vi "multipart_upload.initialize_upload.vi"() -> ()   [LabVIEW 2020, in "Nominal Client.lvclass"]
uses:
  Nominal Client.lvclass
  <vilib>/addons/_JKI.lib/REST Client/classes/REST Client/REST Client.lvclass
  upload.part_core.vi
  Nominal Client.lvclass/Nominal Client.ctl
  Nominal Client MultiPart Upload/Multipart Upload.lvclass
panel:
  out "output cluster":T1
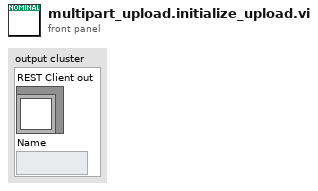
[diagram p1: front panel]
types:
  T1 = cluster{"REST Client out":refnum<class "REST Client.lvclass">, "Name":string}
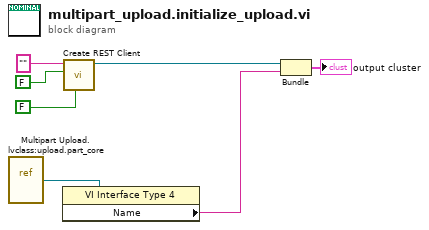
[diagram p0: block diagram]
diagram:
  n1 = vi-ref "Multipart Upload.lvclass:upload.part_core.vi"() -> (w4:refnum<vi>)
  n2 = property class="VI Interface Type 4"(reference=w4) -> ("Name"=w2:string)  [unwired: 1 in, 2 out]
  n3 = call <vilib>:"Create REST Client.vi"("Verify Server(true)"=FALSE, "Escape URLs (true)"=FALSE, "Base URL"="") -> ("REST Client out"=w3:refnum<class "REST Client.lvclass">)  [unwired: 7 in, 1 out]
  n4 = Bundle("REST Client out"=w3, "Name"=w2) -> (→"output cluster":T1)  [unwired: 1 in]
